vi "Tool_Unicode Update Table Data.vi"(5 "Interpret as Unicode (T)":bool=TRUE, 6 "error in (no error)":errorcluster, 8 "Data[]":string[][](array[string]), 9 "Table Ref":refnum<vi>) -> (0 "error out":errorcluster, 3 "Table Ref":refnum<vi>)   [LabVIEW 2009]
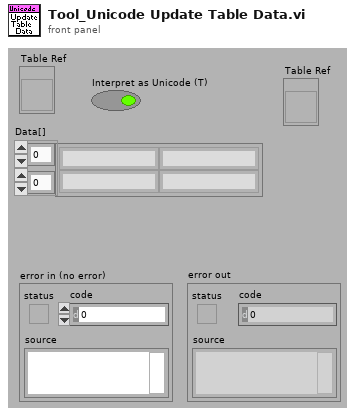
[diagram p1: front panel]
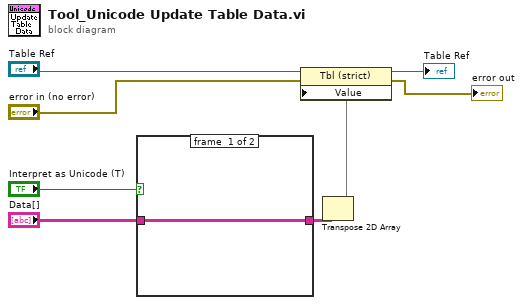
[diagram p0: block diagram]
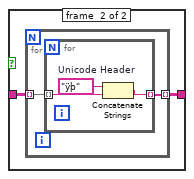
[diagram p2: hidden frame]
diagram:
  n1 = case shown="False" "Interpret as Unicode (T)" {
    tunnel: "Data[]" -> [w9 w11]
    tunnel: [w9 w10] -> w6
    frame #0 {
    }
    frame #1 {
      n2 = for {
        tunnel: w11 -> [w13] mode=indexing
        tunnel: [w12] -> w10 mode=indexing
        n3 = for {
          tunnel: w13 -> [w16] mode=indexing
          tunnel: [w15] -> w12 mode=indexing
          w14 = "ÿþ"  # Unicode Header
          n4 = Concatenate Strings(w14, w16) -> (w15:string)
        }
      }
    }
  }
  n5 = Transpose 2D Array(2D array=w6) -> (transposed array=w1:string[][])
  n6 = property class="Tbl (strict)"(reference="Table Ref", error in="error in (no error)", "Value"=w1) -> (reference out=→"Table Ref":refnum<vi>, error out=→"error out":errorcluster)
